vi "Walking man.vi"() -> ()   [LabVIEW 2011]
panel:
  out "Boolean 56":bool
  out "Boolean 55":bool
  out "Boolean 54":bool
  out "Boolean 53":bool
  out "Boolean 52":bool
  out "Boolean 51":bool
  out "Boolean 50":bool
  out "Boolean 49":bool
  out "Boolean 48":bool
  out "Boolean 47":bool
  out "Boolean 46":bool
  out "Boolean 45":bool
  out "Boolean 44":bool
  out "Boolean 43":bool
  out "Boolean 42":bool
  out "Boolean 41":bool
  out "Boolean 40":bool
  out "Boolean 39":bool
  out "Boolean 38":bool
  out "Boolean 37":bool
  out "Boolean 36":bool
  out "Boolean 35":bool
  out "Boolean 34":bool
  out "Boolean 33":bool
  out "Boolean 32":bool
  out "Boolean 31":bool
  out "Boolean 30":bool
  out "Boolean 29":bool
  out "Boolean 28":bool
  out "Boolean 27":bool
  out "Boolean 26":bool
  out "Boolean 25":bool
  out "Boolean 24":bool
  out "Boolean 23":bool
  out "Boolean 22":bool
  out "Boolean 21":bool
  out "Boolean 20":bool
  out "Boolean 19":bool
  out "Boolean 18":bool
  out "Boolean 17":bool
  out "Boolean 16":bool
  out "Boolean 15":bool
  out "Boolean 14":bool
  out "Boolean 13":bool
  out "Boolean 12":bool
  out "Boolean 11":bool
  out "Boolean 10":bool
  out "Boolean 9":bool
  out "Boolean 8":bool
  out "Boolean 7":bool
  out "Boolean 6":bool
  out "Boolean 5":bool
  out "Boolean 4":bool
  out "Boolean 3":bool
  out "Boolean 2":bool
  out "Boolean":bool
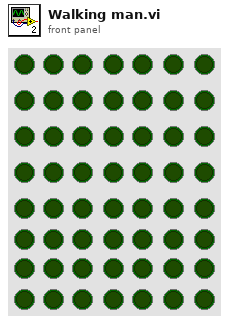
[diagram p1: front panel]
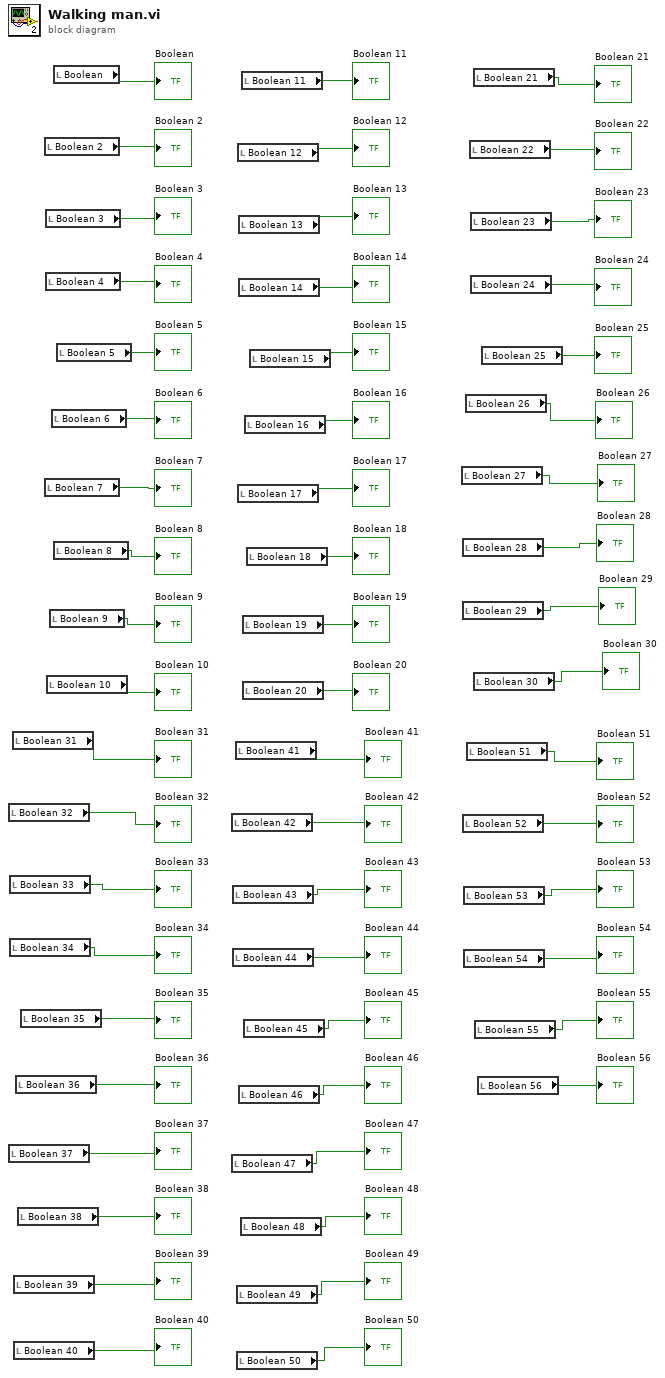
[diagram p0: block diagram]
diagram:
  n1 = local read "Boolean 32"() -> (→"Boolean 32":bool)
  n2 = local read "Boolean 37"() -> (→"Boolean 37":bool)
  n3 = local read "Boolean 33"() -> (→"Boolean 33":bool)
  n4 = local read "Boolean 34"() -> (→"Boolean 34":bool)
  n5 = local read "Boolean 31"() -> (→"Boolean 31":bool)
  n6 = local read "Boolean 39"() -> (→"Boolean 39":bool)
  n7 = local read "Boolean 40"() -> (→"Boolean 40":bool)
  n8 = local read "Boolean 36"() -> (→"Boolean 36":bool)
  n9 = local read "Boolean 38"() -> (→"Boolean 38":bool)
  n10 = local read "Boolean 35"() -> (→"Boolean 35":bool)
  n11 = local read "Boolean 2"() -> (→"Boolean 2":bool)
  n12 = local read "Boolean 7"() -> (→"Boolean 7":bool)
  n13 = local read "Boolean 3"() -> (→"Boolean 3":bool)
  n14 = local read "Boolean 4"() -> (→"Boolean 4":bool)
  n15 = local read "Boolean 10"() -> (→"Boolean 10":bool)
  n16 = local read "Boolean 9"() -> (→"Boolean 9":bool)
  n17 = local read "Boolean 6"() -> (→"Boolean 6":bool)
  n18 = local read "Boolean"() -> (→"Boolean":bool)
  n19 = local read "Boolean 8"() -> (→"Boolean 8":bool)
  n20 = local read "Boolean 5"() -> (→"Boolean 5":bool)
  n21 = local read "Boolean 42"() -> (→"Boolean 42":bool)
  n22 = local read "Boolean 47"() -> (→"Boolean 47":bool)
  n23 = local read "Boolean 43"() -> (→"Boolean 43":bool)
  n24 = local read "Boolean 44"() -> (→"Boolean 44":bool)
  n25 = local read "Boolean 41"() -> (→"Boolean 41":bool)
  n26 = local read "Boolean 49"() -> (→"Boolean 49":bool)
  n27 = local read "Boolean 50"() -> (→"Boolean 50":bool)
  n28 = local read "Boolean 12"() -> (→"Boolean 12":bool)
  n29 = local read "Boolean 17"() -> (→"Boolean 17":bool)
  n30 = local read "Boolean 13"() -> (→"Boolean 13":bool)
  n31 = local read "Boolean 14"() -> (→"Boolean 14":bool)
  n32 = local read "Boolean 46"() -> (→"Boolean 46":bool)
  n33 = local read "Boolean 48"() -> (→"Boolean 48":bool)
  n34 = local read "Boolean 11"() -> (→"Boolean 11":bool)
  n35 = local read "Boolean 19"() -> (→"Boolean 19":bool)
  n36 = local read "Boolean 20"() -> (→"Boolean 20":bool)
  n37 = local read "Boolean 45"() -> (→"Boolean 45":bool)
  n38 = local read "Boolean 16"() -> (→"Boolean 16":bool)
  n39 = local read "Boolean 18"() -> (→"Boolean 18":bool)
  n40 = local read "Boolean 15"() -> (→"Boolean 15":bool)
  n41 = local read "Boolean 27"() -> (→"Boolean 27":bool)
  n42 = local read "Boolean 28"() -> (→"Boolean 28":bool)
  n43 = local read "Boolean 29"() -> (→"Boolean 29":bool)
  n44 = local read "Boolean 52"() -> (→"Boolean 52":bool)
  n45 = local read "Boolean 53"() -> (→"Boolean 53":bool)
  n46 = local read "Boolean 54"() -> (→"Boolean 54":bool)
  n47 = local read "Boolean 26"() -> (→"Boolean 26":bool)
  n48 = local read "Boolean 51"() -> (→"Boolean 51":bool)
  n49 = local read "Boolean 22"() -> (→"Boolean 22":bool)
  n50 = local read "Boolean 23"() -> (→"Boolean 23":bool)
  n51 = local read "Boolean 24"() -> (→"Boolean 24":bool)
  n52 = local read "Boolean 21"() -> (→"Boolean 21":bool)
  n53 = local read "Boolean 30"() -> (→"Boolean 30":bool)
  n54 = local read "Boolean 55"() -> (→"Boolean 55":bool)
  n55 = local read "Boolean 56"() -> (→"Boolean 56":bool)
  n56 = local read "Boolean 25"() -> (→"Boolean 25":bool)
